vi "生成word报表.vi"(0 "Array输入":refnum<vi>, 1 "产品序号":string, 2 "标注图":T1(plugin-control), 3 "缺陷项目":u16(ring) items=["分层、孔洞或脱粘", "弥散性缺陷"], 4 "测试人":string, 5 "部位":string, 6 "类型":string, 7 "产品序号":string, 8 "原图":T1(plugin-control) caption="Original Image") -> (14 "报告生成路径":path)   [LabVIEW 2018]
uses:
  <vilib>/Utility/NIReport.llb/Report Type.ctl
  <vilib>/Utility/NIReport.llb/Append Report Text (str wrap).vi
  <vilib>/addons/_office/word.llb/Word Edit Cell ([dbl]).vi
  <vilib>/addons/_office/word.llb/Word Edit Cell (str).vi
  <vilib>/Utility/NIReport.llb/Append Image to Report (path wrap).vi
  <vilib>/Utility/NIReport.llb/Append Report Text (num wrap).vi
  <vilib>/Utility/NIReport.llb/NI_report.lvclass
  <vilib>/addons/_office/NI_ReportGenerationToolkit.lvlib
  <vilib>/Utility/NIReport.llb/Word/NI_Word.lvclass
  <vilib>/Utility/NIReport.llb/NI_ReportGenerationCore.lvlib
panel:
  out "累计缺陷占比":dbl
  out "值":dbl[][](array[numeric])
  out "Z值":dbl[](array[numeric])
  out "缺陷个数":i32
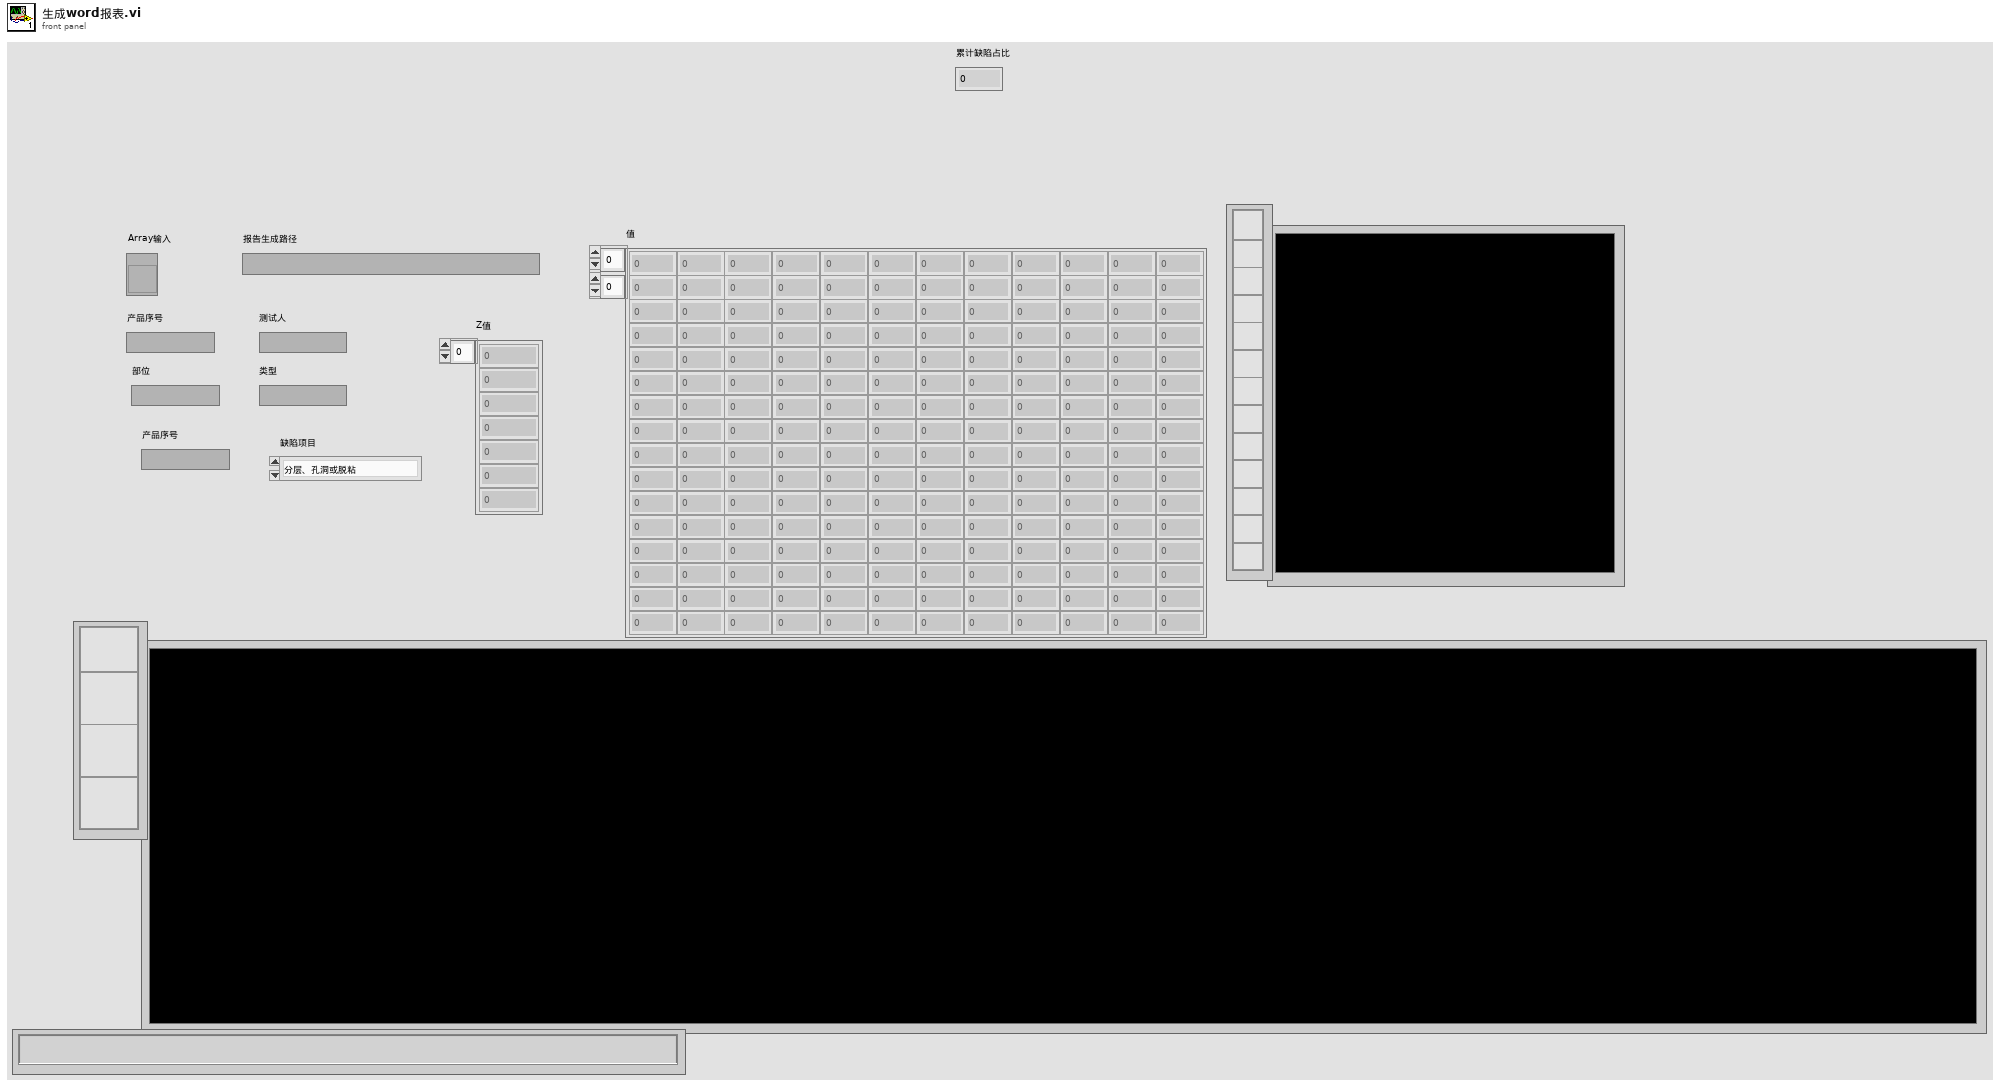
[diagram p1: front panel]
types:
  T1 = typedef "IMAQ Image.ctl" = refnum<image>
  T2 = cluster{"position (Excel)":cluster{"row":i32, "column":i32}, "name (Excel)":string, "bookmark (Word)":string}
  T3 = typedef "NI_ReportGenerationCore.lvlib/Report Type.ctl" = enum16{"HTML", "Word", "Excel"}
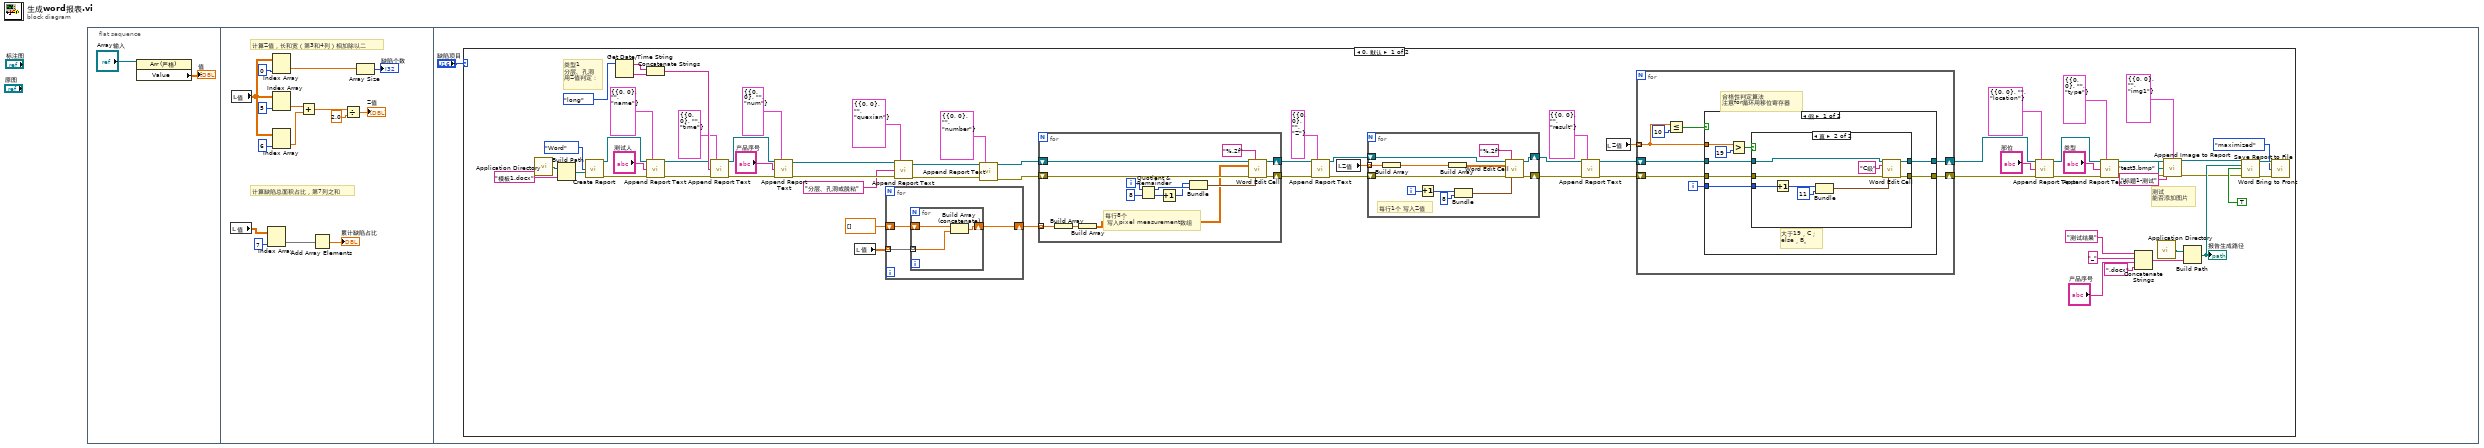
[diagram p0: block diagram]
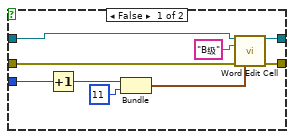
[diagram p2: hidden frame]
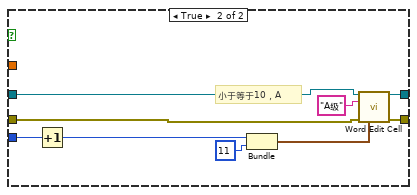
[diagram p3: hidden frame]
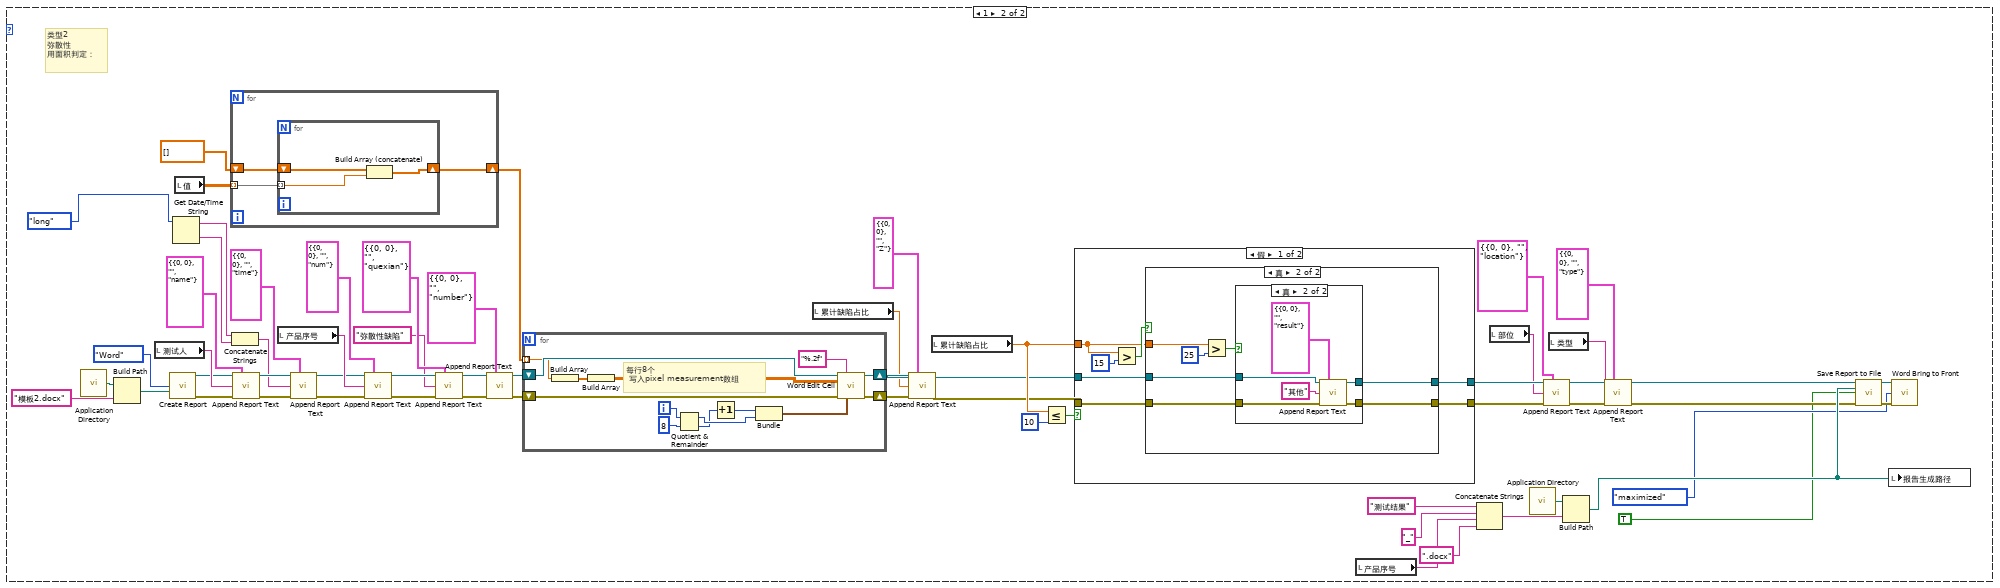
[diagram p4: hidden frame]
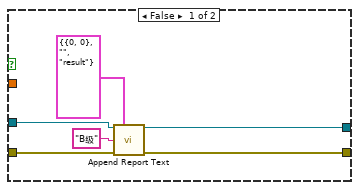
[diagram p5: hidden frame]
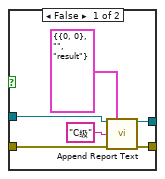
[diagram p6: hidden frame]
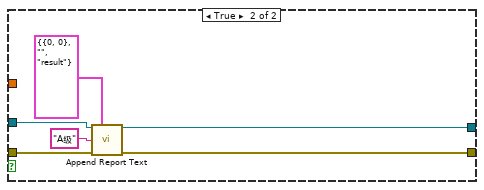
[diagram p7: hidden frame]
diagram:
  n1 = flat-sequence {
    frame #0 {
      n2 = property class="Arr (严格)"(reference="Array输入") -> ("Value"=→"值":dbl[][])  [unwired: 1 in, 2 out]
    }
    frame #1 {
      # "计算缺陷总面积占比，第7列之和"
      # "计算Z值，长和宽（第3和4列）相加除以二"
      n3 = local read "值"() -> (w6:dbl[][])
      n4 = local read "值"() -> (w17:dbl[][])
      n5 = Index Array(array=w6, index (col)=7 ("禁用的索引 (列)")) -> (element=w4:dbl[])  [unwired: 1 in]
      n6 = Index Array(array=w17, index (col)=0 ("禁用的索引 (列)")) -> (element=w14:dbl[])  [unwired: 1 in]
      n7 = Index Array(array=w17, index (col)=5 ("索引")) -> (element=w11:dbl[])  [unwired: 1 in]
      n8 = Index Array(array=w17, index (col)=6 ("索引")) -> (element=w12:dbl[])  [unwired: 1 in]
      n9 = Add(x=w11, y=w12) -> (x+y=w13:dbl[])
      n10 = Add Array Elements(numeric array=w4) -> (sum=→"累计缺陷占比":dbl)
      n11 = Divide(x=w13, y=2.0) -> (x/y=→"Z值":dbl[])
      n12 = Array Size(array=w14) -> (size(s)=→"缺陷个数":i32)
    }
    frame #2 {
      n13 = case shown="0, 默认" "缺陷项目" {
        frame 0, Default {
          # "测试\n能否添加图片"
          # "类型1\n分层、孔洞\n用Z值判定："
          n14 = call <vilib>:"Application Directory.vi"() -> ("Application Directory"=w64:path)
          n15 = Build Path(base path=w64, name or relative path="模板1.docx") -> (appended path=w63:path)
          n16 = call <vilib>:"Create Report.vi"("report type"=Report_Type."Word" ("Report Type"), "template (empty)"=w63) -> ("report out"=w56:refnum<class "NI_report.lvclass">, "error out"=w53:errorcluster)  [unwired: 12 in]
          n17 = Get Date/Time String(date format (0)=enum16{"short", "long", "abbreviated"}."long" ("日期格式(0)")) -> (date string=w62:string, time string=w60:string)  [unwired: 2 in]
          n18 = Concatenate Strings(w62, w60) -> (w61:string)
          n19 = call-poly <vilib>:"Append Report Text.vi"("report in"=w56, "MS Office parameters"=T2 {"position (Excel)"={"row"=0, "column"=0}, "name (Excel)"="", "bookmark (Word)"="name"}, "text"="测试人", "error in (no error)"=w53) -> ("report out"=w55:refnum<class "NI_report.lvclass">, "error out"=w54:errorcluster)  [unwired: 8 in, 2 out]
          n20 = call-poly <vilib>:"Append Report Text.vi"("report in"=w55, "MS Office parameters"=T2 {"position (Excel)"={"row"=0, "column"=0}, "name (Excel)"="", "bookmark (Word)"="time"}, "text"=w61, "error in (no error)"=w54) -> ("report out"=w59:refnum<class "NI_report.lvclass">, "error out"=w58:errorcluster)  [unwired: 8 in, 2 out]
          n21 = call-poly <vilib>:"Append Report Text.vi"("report in"=w59, "MS Office parameters"=T2 {"position (Excel)"={"row"=0, "column"=0}, "name (Excel)"="", "bookmark (Word)"="num"}, "text"="产品序号", "error in (no error)"=w58) -> ("report out"=w28:refnum<class "NI_report.lvclass">, "error out"=w27:errorcluster)  [unwired: 8 in, 2 out]
          n22 = local read "值"() -> (w68:dbl[][])
          n23 = for {
            tunnel: w68 -> [w145] mode=indexing
            shift-right: [w143] -> w57
            shift-left: dbl[] [] ("元素") -> [w144]
            n24 = for {
              tunnel: w145 -> [w148] mode=indexing
              shift-right: [w146] -> w143
              shift-left: w144 -> [w147]
              n25 = Build Array (concatenate)(w147, w148) -> (w146:dbl[])
            }
          }
          n26 = call-poly <vilib>:"Append Report Text.vi"("report in"=w28, "MS Office parameters"=T2 {"position (Excel)"={"row"=0, "column"=0}, "name (Excel)"="", "bookmark (Word)"="quexian"}, "text"="分层、孔洞或脱粘", "error in (no error)"=w27) -> ("report out"=w30:refnum<class "NI_report.lvclass">, "error out"=w29:errorcluster)  [unwired: 8 in, 2 out]
          n27 = call-poly <vilib>:"Append Report Text.vi"("report in"=w30, "MS Office parameters"=T2 {"position (Excel)"={"row"=0, "column"=0}, "name (Excel)"="", "bookmark (Word)"="number"}, "error in (no error)"=w29) -> ("report out"=w66:refnum<class "NI_report.lvclass">, "error out"=w65:errorcluster)  [unwired: 9 in, 2 out]
          n28 = for {
            shift-right: [w162] -> w49
            shift-left: w66 -> [w157]
            shift-right: [w161] -> w87
            shift-left: w65 -> [w156]
            tunnel: w57 -> [w150] mode=indexing
            i -> [w158]
            # "每行8个\n 写入pixel measurement数组"
            n29 = Build Array(w150) -> (w152:dbl[])
            n30 = Build Array(w152) -> (w151:dbl[][])
            n31 = Quotient & Remainder(x=w158, y=8) -> (x-y*floor(x/y)=w155:i32, floor(x/y)=w154:i32)
            n32 = Increment(x=w154) -> (x+1=w153:i32)
            n33 = Bundle(w153, w155) -> (w160:cluster{i32, i32})  [unwired: 1 in]
            n34 = call-poly <vilib>:"Word Edit Cell.vi"("report in"=w157, "format string (%.3f)"="%.2f", "value"=w151, "error in (no error)"=w156, "start (0, 0)"=w160) -> ("report out"=w162:refnum<class "NI_report.lvclass">, "error out"=w161:errorcluster)  [unwired: 9 in]
          }
          n35 = call-poly <vilib>:"Append Report Text.vi"("report in"=w49, "MS Office parameters"=T2 {"position (Excel)"={"row"=0, "column"=0}, "name (Excel)"="", "bookmark (Word)"="Z"}, "error in (no error)"=w87) -> ("report out"=w76:refnum<class "NI_report.lvclass">, "error out"=w75:errorcluster)  [unwired: 9 in, 2 out]
          n36 = local read "Z值"() -> (w69:dbl[])
          n37 = for {
            shift-right: [w142] -> w72
            shift-left: w76 -> [w139]
            shift-right: [w141] -> w71
            shift-left: w75 -> [w138]
            tunnel: w69 -> [w134] mode=indexing
            i -> [w132]
            # "每行1个 写入Z值"
            n38 = Build Array(w134) -> (w136:dbl[])
            n39 = Increment(x=w132) -> (x+1=w137:i32)
            n40 = Build Array(w136) -> (w135:dbl[][])
            n41 = Bundle(w137, "y"=8) -> (w140:cluster{i32, "y":i32})  [unwired: 1 in]
            n42 = call-poly <vilib>:"Word Edit Cell.vi"("report in"=w139, "format string (%.3f)"="%.2f", "value"=w135, "error in (no error)"=w138, "start (0, 0)"=w140) -> ("report out"=w142:refnum<class "NI_report.lvclass">, "error out"=w141:errorcluster)  [unwired: 9 in]
          }
          n43 = call-poly <vilib>:"Append Report Text.vi"("report in"=w72, "MS Office parameters"=T2 {"position (Excel)"={"row"=0, "column"=0}, "name (Excel)"="", "bookmark (Word)"="result"}, "error in (no error)"=w71) -> ("report out"=w73:refnum<class "NI_report.lvclass">, "error out"=w74:errorcluster)  [unwired: 9 in, 2 out]
          n44 = local read "Z值"() -> (w70:dbl[])
          n45 = for {
            shift-right: [w89] -> w50
            shift-left: w73 -> [w92]
            shift-right: [w90] -> w51
            shift-left: w74 -> [w91]
            tunnel: w70 -> [w88] mode=indexing
            i -> [w93]
            # "合格性判定算法\n注意for循环用移位寄存器"
            n46 = Less Or Equal?(x=w88, y=10) -> (x <= y?=w94:bool)
            n47 = case shown="假" w94 {
              tunnel: w93 -> [w100 w128]
              tunnel: w92 -> [w99 w127]
              tunnel: w91 -> [w98 w126]
              tunnel: [w96 w125] -> w90
              tunnel: [w97 w124] -> w89
              tunnel: w88 -> [w103 _]
              frame False {
                # "大于19，C；\nelse，B。"
                n48 = Greater?(x=w103, y=19) -> (0:w101:bool)
                n49 = case shown="真" w101 {
                  tunnel: w100 -> [w104 w117]
                  tunnel: w99 -> [w108 w116]
                  tunnel: w98 -> [w107 w115]
                  tunnel: [w106 w114] -> w97
                  tunnel: [w105 w113] -> w96
                  frame False {
                    n50 = Increment(x=w104) -> (x+1=w112:i32)
                    n51 = Bundle(w112, "y"=11) -> (w111:cluster{i32, "y":i32})  [unwired: 1 in]
                    n52 = call-poly <vilib>:"Word Edit Cell.vi"("report in"=w108, "value"="B级", "error in (no error)"=w107, "start (0, 0)"=w111) -> ("report out"=w106:refnum<class "NI_report.lvclass">, "error out"=w105:errorcluster)  [unwired: 10 in]
                  }
                  frame True {
                    n53 = Increment(x=w117) -> (x+1=w121:i32)
                    n54 = Bundle(w121, "y"=11) -> (w120:cluster{i32, "y":i32})  [unwired: 1 in]
                    n55 = call-poly <vilib>:"Word Edit Cell.vi"("report in"=w116, "value"="C级", "error in (no error)"=w115, "start (0, 0)"=w120) -> ("report out"=w114:refnum<class "NI_report.lvclass">, "error out"=w113:errorcluster)  [unwired: 10 in]
                  }
                }
              }
              frame True {
                # "小于等于10，A"
                n56 = Increment(x=w128) -> (x+1=w130:i32)
                n57 = Bundle(w130, "y"=11) -> (w122:cluster{i32, "y":i32})  [unwired: 1 in]
                n58 = call-poly <vilib>:"Word Edit Cell.vi"("report in"=w127, "value"="A级", "error in (no error)"=w126, "start (0, 0)"=w122) -> ("report out"=w124:refnum<class "NI_report.lvclass">, "error out"=w125:errorcluster)  [unwired: 10 in]
              }
            }
          }
          n59 = call-poly <vilib>:"Append Report Text.vi"("report in"=w50, "MS Office parameters"=T2 {"position (Excel)"={"row"=0, "column"=0}, "name (Excel)"="", "bookmark (Word)"="location"}, "text"="部位", "error in (no error)"=w51) -> ("report out"=w84:refnum<class "NI_report.lvclass">, "error out"=w83:errorcluster)  [unwired: 8 in, 2 out]
          n60 = call-poly <vilib>:"Append Report Text.vi"("report in"=w84, "MS Office parameters"=T2 {"position (Excel)"={"row"=0, "column"=0}, "name (Excel)"="", "bookmark (Word)"="type"}, "text"="类型", "error in (no error)"=w83) -> ("report out"=w25:refnum<class "NI_report.lvclass">, "error out"=w22:errorcluster)  [unwired: 8 in, 2 out]
          n61 = Concatenate Strings("测试结果" ("字符串"), "_" ("名称或相对路径"), "产品序号", ".docx" ("名称或相对路径")) -> (w80:string)
          n62 = call <vilib>:"Application Directory.vi"() -> ("Application Directory"=w81:path)
          n63 = call-poly <vilib>:"Append Image to Report.vi"("report in"=w25, "MS Office parameters"=T2 {"position (Excel)"={"row"=0, "column"=0}, "name (Excel)"="", "bookmark (Word)"="img1"}, "path or URL of image"=path "test3.bmp", "caption or alternative string"="标题1-测试", "error in (no error)"=w22) -> ("report out"=w24:refnum<class "NI_report.lvclass">, "error out"=w23:errorcluster)  [unwired: 7 in, 2 out]
          n64 = Build Path(base path=w81, name or relative path=w80) -> (appended path=w82:path)
          "报告生成路径" <- w82
          n65 = call-dynamic "Save Report to File.vi"("report in"=w24, "report file path"=w82, "prompt to replace? (F)"=TRUE, "error in (no error)"=w23) -> ("report out"=w79:refnum<class "NI_report.lvclass">, "error out"=w78:errorcluster)  [unwired: 10 in]
          n66 = call <vilib>:"Word Bring to Front.vi"("report in"=w79, "window state (maximized)"=enum16{"maximized", "minimized", "normal"}."maximized", "error in (no error)"=w78) -> ()  [unwired: 11 in, 2 out]
        }
        frame 1 {
          # "类型2\n弥散性\n用面积判定："
          n67 = call <vilib>:"Application Directory.vi"() -> ("Application Directory"=w194:path)
          n68 = Build Path(base path=w194, name or relative path="模板2.docx") -> (appended path=w195:path)
          n69 = local read "测试人"() -> (w211:string)
          n70 = call <vilib>:"Create Report.vi"("report type"=Report_Type."Word" ("Report Type"), "template (empty)"=w195) -> ("report out"=w202:refnum<class "NI_report.lvclass">, "error out"=w205:errorcluster)  [unwired: 12 in]
          n71 = Get Date/Time String(date format (0)=enum16{"short", "long", "abbreviated"}."long" ("日期格式(0)")) -> (date string=w196:string, time string=w198:string)  [unwired: 2 in]
          n72 = local read "值"() -> (w191:dbl[][])
          n73 = for {
            tunnel: w191 -> [w264] mode=indexing
            shift-right: [w262] -> w201
            shift-left: dbl[] [] ("元素") -> [w263]
            n74 = for {
              tunnel: w264 -> [w267] mode=indexing
              shift-right: [w265] -> w262
              shift-left: w263 -> [w266]
              n75 = Build Array (concatenate)(w266, w267) -> (w265:dbl[])
            }
          }
          n76 = Concatenate Strings(w196, w198) -> (w197:string)
          n77 = call-poly <vilib>:"Append Report Text.vi"("report in"=w202, "MS Office parameters"=T2 {"position (Excel)"={"row"=0, "column"=0}, "name (Excel)"="", "bookmark (Word)"="name"}, "text"=w211, "error in (no error)"=w205) -> ("report out"=w203:refnum<class "NI_report.lvclass">, "error out"=w204:errorcluster)  [unwired: 8 in, 2 out]
          n78 = local read "产品序号"() -> (w212:string)
          n79 = call-poly <vilib>:"Append Report Text.vi"("report in"=w203, "MS Office parameters"=T2 {"position (Excel)"={"row"=0, "column"=0}, "name (Excel)"="", "bookmark (Word)"="time"}, "text"=w197, "error in (no error)"=w204) -> ("report out"=w199:refnum<class "NI_report.lvclass">, "error out"=w200:errorcluster)  [unwired: 8 in, 2 out]
          n80 = call-poly <vilib>:"Append Report Text.vi"("report in"=w199, "MS Office parameters"=T2 {"position (Excel)"={"row"=0, "column"=0}, "name (Excel)"="", "bookmark (Word)"="num"}, "text"=w212, "error in (no error)"=w200) -> ("report out"=w209:refnum<class "NI_report.lvclass">, "error out"=w210:errorcluster)  [unwired: 8 in, 2 out]
          n81 = call-poly <vilib>:"Append Report Text.vi"("report in"=w209, "MS Office parameters"=T2 {"position (Excel)"={"row"=0, "column"=0}, "name (Excel)"="", "bookmark (Word)"="quexian"}, "text"="弥散性缺陷", "error in (no error)"=w210) -> ("report out"=w207:refnum<class "NI_report.lvclass">, "error out"=w208:errorcluster)  [unwired: 8 in, 2 out]
          n82 = call-poly <vilib>:"Append Report Text.vi"("report in"=w207, "MS Office parameters"=T2 {"position (Excel)"={"row"=0, "column"=0}, "name (Excel)"="", "bookmark (Word)"="number"}, "error in (no error)"=w208) -> ("report out"=w192:refnum<class "NI_report.lvclass">, "error out"=w193:errorcluster)  [unwired: 9 in, 2 out]
          n83 = for {
            shift-right: [w281] -> w206
            shift-left: w192 -> [w276]
            shift-right: [w280] -> w182
            shift-left: w193 -> [w275]
            tunnel: w201 -> [w269] mode=indexing
            i -> [w277]
            # "每行8个\n 写入pixel measurement数组"
            n84 = Build Array(w269) -> (w271:dbl[])
            n85 = Build Array(w271) -> (w270:dbl[][])
            n86 = Quotient & Remainder(x=w277, y=8) -> (x-y*floor(x/y)=w274:i32, floor(x/y)=w273:i32)
            n87 = Increment(x=w273) -> (x+1=w272:i32)
            n88 = Bundle(w272, w274) -> (w279:cluster{i32, i32})  [unwired: 1 in]
            n89 = call-poly <vilib>:"Word Edit Cell.vi"("report in"=w276, "format string (%.3f)"="%.2f", "value"=w270, "error in (no error)"=w275, "start (0, 0)"=w279) -> ("report out"=w281:refnum<class "NI_report.lvclass">, "error out"=w280:errorcluster)  [unwired: 9 in]
          }
          n90 = local read "累计缺陷占比"() -> (w217:dbl)
          n91 = call-poly <vilib>:"Append Report Text.vi"("report in"=w206, "MS Office parameters"=T2 {"position (Excel)"={"row"=0, "column"=0}, "name (Excel)"="", "bookmark (Word)"="Z"}, "text"=w217, "error in (no error)"=w182) -> ("report out"=w218:refnum<class "NI_report.lvclass">, "error out"=w219:errorcluster)  [unwired: 8 in, 2 out]
          n92 = local read "累计缺陷占比"() -> (w223:dbl)
          n93 = Less Or Equal?(x=w223, y=10) -> (x <= y?=w222:bool)
          n94 = case shown="假" w222 {
            tunnel: w218 -> [w228 w259]
            tunnel: w219 -> [w226 w258]
            tunnel: [w225 w257] -> w220
            tunnel: [w227 w256] -> w221
            tunnel: w223 -> [w224 _]
            frame False {
              n95 = Greater?(x=w224, y=15) -> (0:w229:bool)
              n96 = case shown="真" w229 {
                tunnel: w228 -> [w234 w240]
                tunnel: [w233 w237] -> w227
                tunnel: w226 -> [w232 w239]
                tunnel: [w231 w238] -> w225
                tunnel: w224 -> [_ w242]
                frame False {
                  n97 = call-poly <vilib>:"Append Report Text.vi"("report in"=w234, "MS Office parameters"=T2 {"position (Excel)"={"row"=0, "column"=0}, "name (Excel)"="", "bookmark (Word)"="result"}, "text"="B级", "error in (no error)"=w232) -> ("report out"=w233:refnum<class "NI_report.lvclass">, "error out"=w231:errorcluster)  [unwired: 8 in, 2 out]
                }
                frame True {
                  n98 = Greater?(x=w242, y=25) -> (0:w241:bool)
                  n99 = case shown="真" w241 {
                    tunnel: w240 -> [w247 w253]
                    tunnel: w239 -> [w246 w252]
                    tunnel: [w245 w251] -> w238
                    tunnel: [w244 w250] -> w237
                    frame False {
                      n100 = call-poly <vilib>:"Append Report Text.vi"("report in"=w247, "MS Office parameters"=T2 {"position (Excel)"={"row"=0, "column"=0}, "name (Excel)"="", "bookmark (Word)"="result"}, "text"="C级", "error in (no error)"=w246) -> ("report out"=w244:refnum<class "NI_report.lvclass">, "error out"=w245:errorcluster)  [unwired: 8 in, 2 out]
                    }
                    frame True {
                      n101 = call-poly <vilib>:"Append Report Text.vi"("report in"=w253, "MS Office parameters"=T2 {"position (Excel)"={"row"=0, "column"=0}, "name (Excel)"="", "bookmark (Word)"="result"}, "text"="其他", "error in (no error)"=w252) -> ("report out"=w250:refnum<class "NI_report.lvclass">, "error out"=w251:errorcluster)  [unwired: 8 in, 2 out]
                    }
                  }
                }
              }
            }
            frame True {
              n102 = call-poly <vilib>:"Append Report Text.vi"("report in"=w259, "MS Office parameters"=T2 {"position (Excel)"={"row"=0, "column"=0}, "name (Excel)"="", "bookmark (Word)"="result"}, "text"="A级", "error in (no error)"=w258) -> ("report out"=w256:refnum<class "NI_report.lvclass">, "error out"=w257:errorcluster)  [unwired: 8 in, 2 out]
            }
          }
          n103 = local read "产品序号"() -> (w215:string)
          n104 = Concatenate Strings("测试结果" ("字符串"), "_" ("名称或相对路径"), w215, ".docx" ("名称或相对路径")) -> (w188:string)
          n105 = local read "部位"() -> (w213:string)
          n106 = call <vilib>:"Application Directory.vi"() -> ("Application Directory"=w187:path)
          n107 = call-poly <vilib>:"Append Report Text.vi"("report in"=w221, "MS Office parameters"=T2 {"position (Excel)"={"row"=0, "column"=0}, "name (Excel)"="", "bookmark (Word)"="location"}, "text"=w213, "error in (no error)"=w220) -> ("report out"=w185:refnum<class "NI_report.lvclass">, "error out"=w186:errorcluster)  [unwired: 8 in, 2 out]
          n108 = local read "类型"() -> (w214:string)
          n109 = Build Path(base path=w187, name or relative path=w188) -> (appended path=w216:path)
          n110 = call-poly <vilib>:"Append Report Text.vi"("report in"=w185, "MS Office parameters"=T2 {"position (Excel)"={"row"=0, "column"=0}, "name (Excel)"="", "bookmark (Word)"="type"}, "text"=w214, "error in (no error)"=w186) -> ("report out"=w184:refnum<class "NI_report.lvclass">, "error out"=w183:errorcluster)  [unwired: 8 in, 2 out]
          n111 = call-dynamic "Save Report to File.vi"("report in"=w184, "report file path"=w216, "prompt to replace? (F)"=TRUE, "error in (no error)"=w183) -> ("report out"=w189:refnum<class "NI_report.lvclass">, "error out"=w190:errorcluster)  [unwired: 10 in]
          n112 = local write "报告生成路径"(w216) -> ()
          n113 = call <vilib>:"Word Bring to Front.vi"("report in"=w189, "window state (maximized)"=enum16{"maximized", "minimized", "normal"}."maximized", "error in (no error)"=w190) -> ()  [unwired: 11 in, 2 out]
        }
      }
    }
  }
